vi "SerialNo.vi"(0 "DB serial number IN":string, 2 "Run uninterrupted?":bool) -> (7 "Continue?":bool)   [LabVIEW 2013]
uses:
  globals/QC_RunInformation.vi
panel:
  in  "DB Serial No.:":string
  in  "Batch No.:":string
  in  "Device Category:":string(combo)="ATLAS18SS"
  in  "Manufacturer:":string(combo)="Hamamatsu"
  in  "Wafer No.:":string
  in  "Cancel":bool
  in  "OK":bool
  # "ATLAS Serial No."
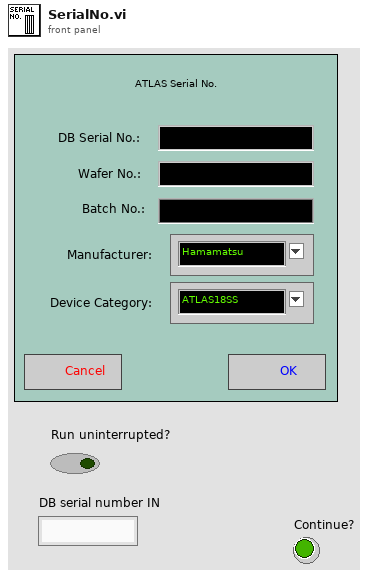
[diagram p1: front panel]
types:
  T1 = cluster{"Institute":string, "Manufacturers":string[], "Devices":string[], "Serialnumbers Lookup DB":string, "Data directory":string, "Backup & screenshot directory":string, "List of known users":string[], "Measurement switch not used":bool, "Measurement Switch":string, "DUT Switch":string, "Rseries IV [MOhm]":string, "Rshunt IV [MOhm]":string, "Rseries CV [MOhm]":string, "DC blocking Cap [µF]":string, "Rseries LCR [MOhm]":string, "Rseries stability [MOhm]":string, "Rshunt stability [MOhm]":string, "Rseries striptest bias [MOhm]":string, "Rseries strip pinhole [MOhm]":string}
  T2 = cluster{"Sensor Serial No.:":string, "Wafer:":string, "Batch:":string, "Manufacturer:":string, "Device Category:":string, "Database Serial No.:":string, "Date Initiated:":string, "Time Initiated:":string, "Test":string, "Probeplan used:":string, "End of Run comment:":string, "User:":string, "Vbias SMU":string, "LCR":string, "Test SMU":string, "Test DMM":string}
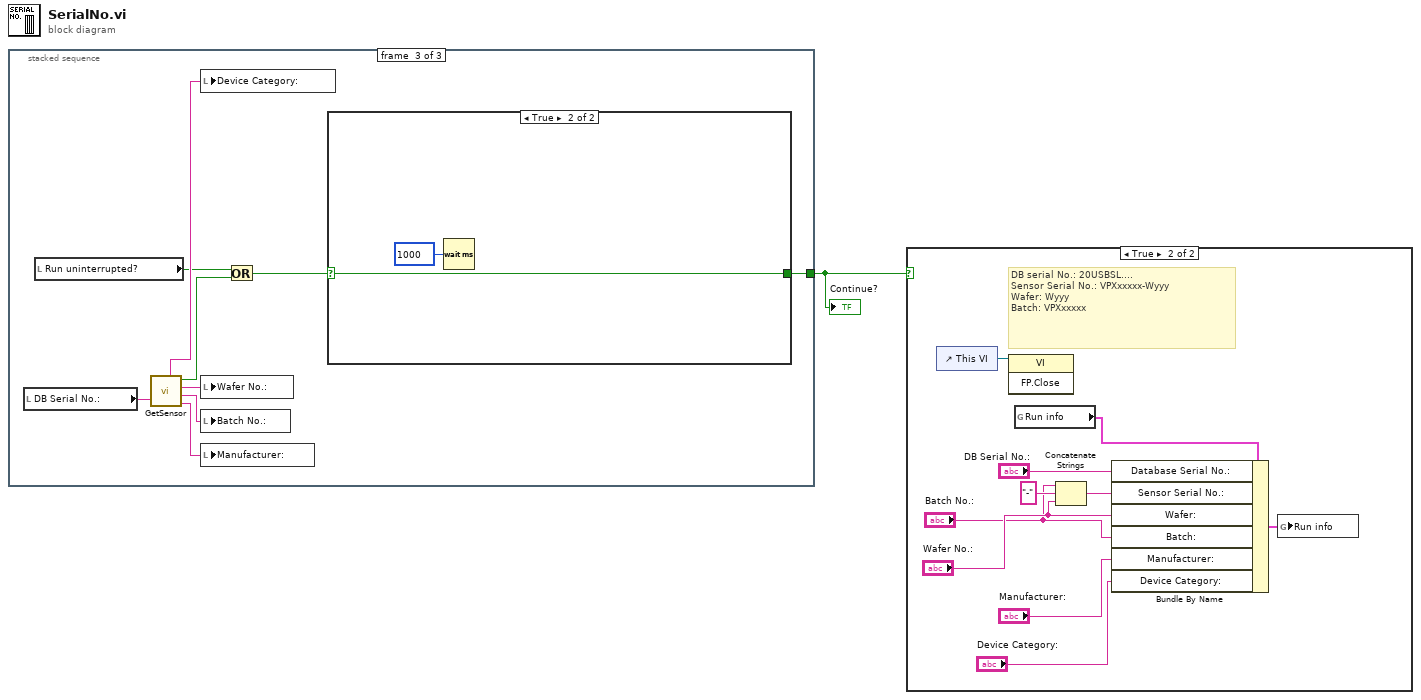
[diagram p0: block diagram]
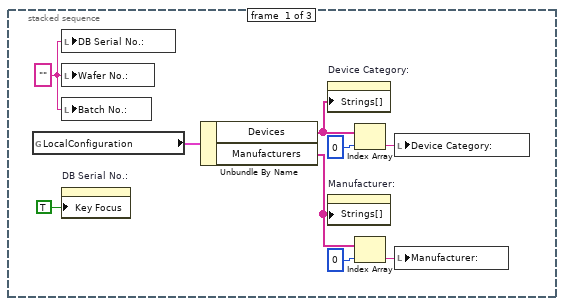
[diagram p2: hidden frame]
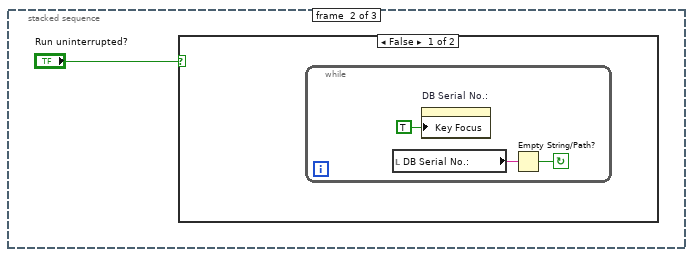
[diagram p3: hidden frame]
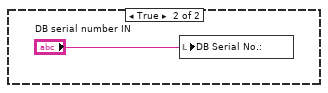
[diagram p4: hidden frame]
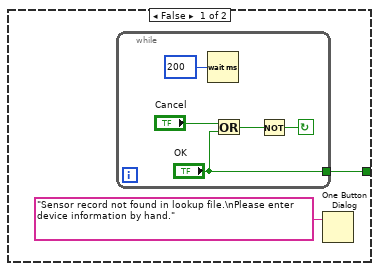
[diagram p5: hidden frame]
diagram:
  n1 = stacked-sequence {
    tunnel: [_ _ w24] -> w1
    frame #0 {
      w10 = ""
      n2 = global read "QC_RunInformation.vi" "LocalConfiguration"() -> (w8:T1)
      n3 = local write "DB Serial No.:"(w10) -> ()
      n4 = local write "Wafer No.:"(w10) -> ()
      n5 = local write "Batch No.:"(w10) -> ()
      n6 = property on="DB Serial No.:" class="Str"("Key Focus"=TRUE) -> ()  [unwired: 2 in, 2 out]
      n7 = Unbundle By Name(w8) -> ("Devices"=w3:string[], "Manufacturers"=w2:string[])
      n8 = property on="Device Category:" class="CmbBox"("Strings[]"=w3) -> ()  [unwired: 2 in, 2 out]
      n9 = property on="Manufacturer:" class="CmbBox"("Strings[]"=w2) -> ()  [unwired: 2 in, 2 out]
      n10 = Index Array(array=w3, index=0) -> (element=w4:string)
      n11 = Index Array(array=w2, index=0) -> (element=w5:string)
      n12 = local write "Device Category:"(w4) -> ()
      n13 = local write "Manufacturer:"(w5) -> ()
    }
    frame #1 {
      n14 = case shown="False" "Run uninterrupted?" {
        frame False {
          n15 = while {
            stop <- w12 continue-if-true
            n16 = local read "DB Serial No.:"() -> (w13:string)
            n17 = property on="DB Serial No.:" class="Str"("Key Focus"=TRUE) -> ()  [unwired: 2 in, 2 out]
            n18 = Empty String/Path?(string/path=w13) -> (empty?=w12:bool)
          }
        }
        frame True {
          n19 = local write "DB Serial No.:"("DB serial number IN") -> ()
        }
      }
    }
    frame #2 {
      n20 = local read "DB Serial No.:"() -> (w19:string)
      n21 = local read "Run uninterrupted?"() -> (w16:bool)
      n22 = call "GetSensor.vi"("DB Serial No. IN"=w19) -> ("Manufacturer"=w22:string, "Batch No."=w21:string, "Wafer No."=w20:string, "Record found?"=w18:bool, "Device Category:"=w23:string)  [unwired: 1 in]
      n23 = local write "Device Category:"(w23) -> ()
      n24 = local write "Wafer No.:"(w20) -> ()
      n25 = local write "Batch No.:"(w21) -> ()
      n26 = local write "Manufacturer:"(w22) -> ()
      n27 = Or(x=w16, y=w18) -> (x .or. y?=w17:bool)
      n28 = case shown="True" w17 {
        selector: w17 -> [_ w33]
        tunnel: [w26 w33] -> w24
        frame False {
          n29 = while {
            tunnel: ["OK"] -> w26
            stop <- w29 continue-if-true
            n30 = Wait (ms)(milliseconds to wait=200) -> ()  [unwired: 1 out]
            n31 = Or(x="Cancel", y="OK") -> (x .or. y?=w30:bool)
            n32 = Not(x=w30) -> (.not. x?=w29:bool)
          }
          n33 = One Button Dialog(message="Sensor record not found in lookup file.\nPlease enter device information by hand.") -> ()  [unwired: 1 in, 1 out]
        }
        frame True {
          n34 = Wait (ms)(milliseconds to wait=1000) -> ()  [unwired: 1 out]
        }
      }
    }
  }
  "Continue?" <- w1
  n35 = case shown="True" w1 {
    frame False {
    }
    frame True {
      # "DB serial No.: 20USBSL....\nSensor Serial No.: VPXxxxxx-Wyyy\nWafer: Wyyy\nBatch: VPXxxxxx"
      n36 = control-ref of="This VI"() -> (w42:refnum<vi>)
      n37 = invoke class="VI" method="FP.Close"(reference=w42) -> ()  [unwired: 2 in, 3 out]
      n38 = global read "QC_RunInformation.vi" "Run info"() -> (w34:T2)
      n39 = Concatenate Strings("Batch No.:", "-", "Wafer No.:") -> (w40:string)
      n40 = Bundle By Name(cluster=w34, "Database Serial No.:"="DB Serial No.:", "Sensor Serial No.:"=w40, "Wafer:"="Wafer No.:", "Batch:"="Batch No.:", "Manufacturer:"="Manufacturer:", "Device Category:"="Device Category:") -> (w43:T2)
      n41 = global write "QC_RunInformation.vi" "Run info"(w43) -> ()
    }
  }
